vi "RC Car.vi"() -> ()   [LabVIEW 2018]
uses:
  <vilib>/LabVIEW Interface for Arduino/Type Defs/Pin Mode.ctl
  <vilib>/LabVIEW Interface for Arduino/LabVIEW Interface for Arduino.lvlib
panel:
  in  "stop":bool
  in  "LEFTWARD":bool
  in  "RIGHTWARD":bool
  in  "BACKWARD":bool
  in  "FORWARD":bool
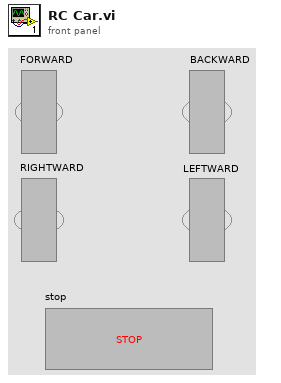
[diagram p1: front panel]
types:
  T1 = typedef "LabVIEW Interface for Arduino.lvlib/Pin Mode.ctl" = enum8{"Input", "Output"}
  T2 = typedef "LabVIEW Interface for Arduino.lvlib/Arduino Resource.ctl" = cluster{"VISA resource":refnum<visa-resource-name>, "Board Type":T3, "Connection Type":enum8{"USB / Serial"}, "Bytes Per Packet (15)":u8}
  T3 = typedef "LabVIEW Interface for Arduino.lvlib/Board Type.ctl" = enum16{"Uno", "Dimuelanove w/Atmega 328", "Mega 2560"}
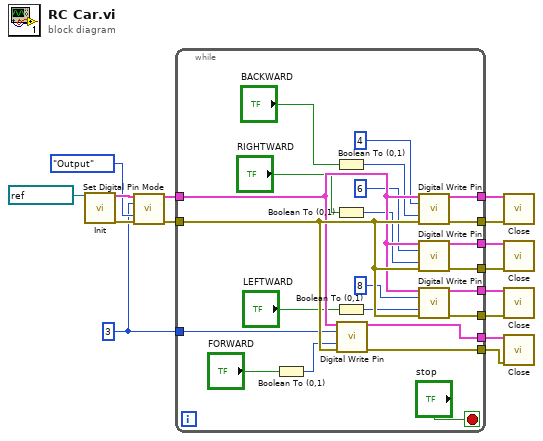
[diagram p0: block diagram]
diagram:
  w1 = u8 3 ("Digital I/O Pin")
  n1 = call <vilib>:"Init.vi"("VISA resource"=refnum<visa-resource-name> "COM 3") -> ("Arduino Resource"=w6:T2, "error out"=w5:errorcluster)  [unwired: 17 in]
  n2 = call <vilib>:"Set Digital Pin Mode.vi"("Arduino Resource"=w6, "Digital I/O Pin"=w1, "Pin Mode (Input)"=Pin_Mode."Output", "error in"=w5) -> ("Arduino Resource"=w3:T2, "error out"=w4:errorcluster)  [unwired: 10 in]
  n3 = while {
    tunnel: [w38] -> w14
    tunnel: [w37] -> w13
    tunnel: [w36] -> w12
    tunnel: [w35] -> w11
    tunnel: [w34] -> w10
    tunnel: [w33] -> w9
    tunnel: [w32] -> w8
    tunnel: [w31] -> w7
    tunnel: w3 -> [w29]
    tunnel: w4 -> [w30]
    tunnel: w1 -> [w16]
    stop <- "stop" stop-if-true
    n4 = Boolean To (0,1)(Boolean="FORWARD") -> (0, 1=w21:i16)
    n5 = Boolean To (0,1)(Boolean="BACKWARD") -> (0, 1=w23:i16)
    n6 = Boolean To (0,1)(Boolean="RIGHTWARD") -> (0, 1=w25:i16)
    n7 = Boolean To (0,1)(Boolean="LEFTWARD") -> (0, 1=w27:i16)
    n8 = call <vilib>:"Digital Write Pin.vi"("Arduino Resource"=w29, "Digital I/O Pin (0)"=w16, "Value (0)"=w21, "error in"=w30) -> ("Arduino Resource"=w38:T2, "error out"=w37:errorcluster)  [unwired: 10 in]
    n9 = call <vilib>:"Digital Write Pin.vi"("Arduino Resource"=w29, "Digital I/O Pin (0)"=u8 4, "Value (0)"=w23, "error in"=w30) -> ("Arduino Resource"=w36:T2, "error out"=w31:errorcluster)  [unwired: 10 in]
    n10 = call <vilib>:"Digital Write Pin.vi"("Arduino Resource"=w29, "Digital I/O Pin (0)"=u8 6, "Value (0)"=w25, "error in"=w30) -> ("Arduino Resource"=w35:T2, "error out"=w32:errorcluster)  [unwired: 10 in]
    n11 = call <vilib>:"Digital Write Pin.vi"("Arduino Resource"=w29, "Digital I/O Pin (0)"=u8 8, "Value (0)"=w27, "error in"=w30) -> ("Arduino Resource"=w34:T2, "error out"=w33:errorcluster)  [unwired: 10 in]
  }
  n12 = call <vilib>:"Close.vi"("Arduino Resource"=w12, "error in"=w7) -> ()  [unwired: 13 in, 1 out]
  n13 = call <vilib>:"Close.vi"("Arduino Resource"=w11, "error in"=w8) -> ()  [unwired: 13 in, 1 out]
  n14 = call <vilib>:"Close.vi"("Arduino Resource"=w10, "error in"=w9) -> ()  [unwired: 13 in, 1 out]
  n15 = call <vilib>:"Close.vi"("Arduino Resource"=w14, "error in"=w13) -> ()  [unwired: 13 in, 1 out]
